vi "Configure IQ Vs Slot Expected Nominal Power.vi"(7 "Expected Nominal Power (0.0)":dbl format="%^.3e", 8 "error in (no error)":errorcluster, 9 "Index (0)":i32, 10 "Instance (1)":i32=1, 11 "VISA resource name":refnum<visa-resource-name>) -> (0 "error out":errorcluster, 3 "VISA resource name out":refnum<visa-resource-name>)   [LabVIEW 2020, in "Rohde&Schwarz CMXP GPRF.lvlib"]
doc: "Defines or queries the expected nominal power of subsweep <Index>.\n\nAttribute:\nRSCMXPGPRF_ATTR_IQ_VS_SLOT_EXPECTED_NOMINAL_POWER\n\nRemote-control command:\nCONFigure:GPRF:MEAS<i>:IQVSlot:LIST:ENPower"
uses:
  <instrlib>/Rohde&Schwarz CMXP GPRF/Rohde&Schwarz CMXP GPRF.lvlib
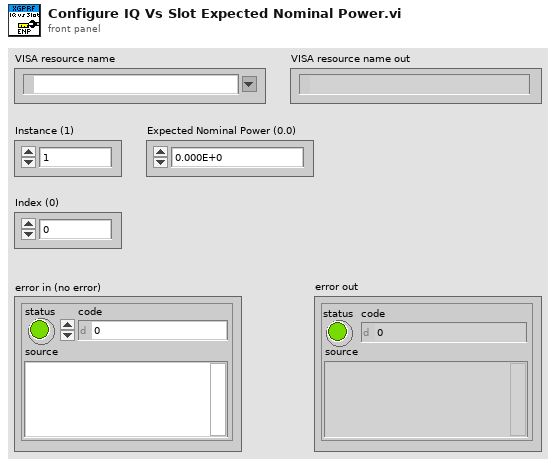
[diagram p1: front panel]
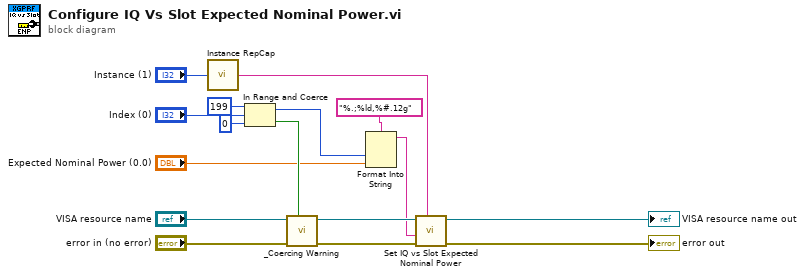
[diagram p0: block diagram]
diagram:
  n1 = call <instrlib>:"Instance RepCap.vi"("Instance in"="Instance (1)") -> ("Instance out"=w5:string)
  n2 = In Range and Coerce(upper limit=199, x="Index (0)", lower limit=0) -> (coerced(x)=w2:i32, In Range?=w6:bool)
  n3 = call <instrlib>:"_Coercing Warning.vi"("In Range?"=w6, "error in (no error)"="error in (no error)", "VISA resource name"="VISA resource name") -> ("error out"=w10:errorcluster, "VISA resource name out"=w9:refnum<visa-resource-name>)  [unwired: 7 in]
  n4 = Format Into String(format string="%.;%ld,%#.12g", w2, "Expected Nominal Power (0.0)") -> (resulting string=w1:string)  [unwired: 2 in, 1 out]
  n5 = call "Set IQ vs Slot Expected Nominal Power"("Repeated Capabilities"=w5, "error in (no error)"=w10, "IQ vs Slot Expected Nominal Power ()"=w1, "instrument handle"=w9) -> ("error out"=→"error out":errorcluster, "instrument handle out"=→"VISA resource name out":refnum<visa-resource-name>)  [unwired: 6 in]
